vi "Interpolate 2D Scattered_Green Function.vi"(0 "X":dbl[](array[numeric]), 5 "Y":dbl[](array[numeric]), 7 "Z":dbl[](array[numeric]), 9 "Xi":dbl[](array[numeric]), 11 "Yi":dbl[](array[numeric])) -> (4 "Zi":dbl[](array[numeric]), 15 "error":i32)   [LabVIEW 2017, in "NI_AAL_Interpolation.lvlib"]
uses:
  <vilib>/gmath/NI_AAL_Interpolation.lvlib
  <vilib>/Analysis/7linalg.llb/Solve Linear Equations (single right hand).vi
  <vilib>/Analysis/baseanly.llb/Real Dot Product.vi
  <vilib>/Analysis/baseanly.llb/Solve Linear Equations By Cholesky.vi
  <vilib>/Analysis/baseanly.llb/Real Matrix to Compact Array.vi
  <vilib>/Analysis/baseanly.llb/Real Compact Tri-Matrix Linear Eqs.vi
  <vilib>/Analysis/7linalg.llb/Solve Linear Eqs (General).vi
  <vilib>/Analysis/7linalg.llb/Solve Linear Eqs (Gen, single right hand).vi
  <vilib>/Analysis/NI_AALPro.lvlib
  <vilib>/Analysis/NI_AALBase.lvlib
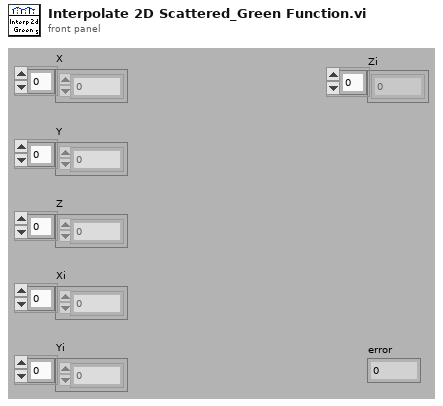
[diagram p1: front panel]
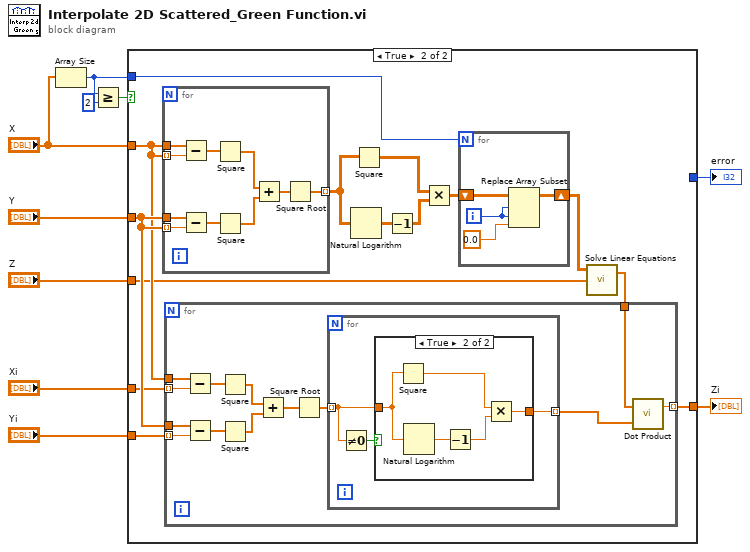
[diagram p0: block diagram]
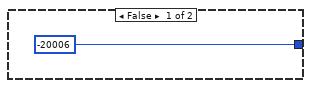
[diagram p2: hidden frame]
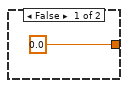
[diagram p3: hidden frame]
diagram:
  n1 = Array Size(array="X") -> (size(s)=w2:i32)
  n2 = Greater Or Equal?(x=w2, y=2) -> (x >= y?=w3:bool)
  n3 = case shown="True" w3 {
    tunnel: "Y" -> [_ w21]
    tunnel: "Xi" -> [_ w20]
    tunnel: "Yi" -> [_ w19]
    tunnel: "X" -> [_ w17]
    tunnel: "Z" -> [_ w16]
    tunnel: [_ w13] -> w6
    tunnel: w2 -> [_ w12]
    tunnel: [-20006 _] -> w1
    frame False {
    }
    frame True {
      n4 = for {
        tunnel: w17 -> [w61]
        tunnel: w21 -> [w60]
        tunnel: w17 -> [w59] mode=indexing
        tunnel: w21 -> [w58] mode=indexing
        tunnel: [w57] -> w25 mode=indexing
        n5 = Subtract(x=w61, y=w59) -> (x-y=w56:dbl[])
        n6 = Subtract(x=w60, y=w58) -> (x-y=w55:dbl[])
        n7 = Square(x=w56) -> (x^2=w53:dbl[])
        n8 = Square(x=w55) -> (x^2=w54:dbl[])
        n9 = Add(x=w53, y=w54) -> (x+y=w52:dbl[])
        n10 = Square Root(x=w52) -> (sqrt(x)=w57:dbl[])
      }
      n11 = Natural Logarithm(1:w25) -> (0:w24:dbl[][])
      n12 = Square(x=w25) -> (x^2=w22:dbl[][])
      n13 = Decrement(x=w24) -> (x-1=w23:dbl[][])
      n14 = Multiply(x=w22, y=w23) -> (x*y=w18:dbl[][])
      n15 = for {
        N: w12 -> [_]
        shift-right: [w28] -> w15
        shift-left: w18 -> [w29]
        i -> [w27]
        n16 = Replace Array Subset(array=w29, new element=0.0 ("new element/subarray"), index (row)=w27, index (col)=w27) -> (w28:dbl[][])
      }
      n17 = call-poly <vilib>:"Solve Linear Equations.vi"("Known Vector"=w16, "Input Matrix"=w15) -> ("Solution Vector"=w14:dbl[])  [unwired: 1 in, 1 out]
      n18 = for {
        tunnel: w17 -> [w42]
        tunnel: w21 -> [w40]
        tunnel: w20 -> [w41] mode=indexing
        tunnel: w19 -> [w39] mode=indexing
        tunnel: w14 -> [w31]
        tunnel: [w30] -> w13 mode=indexing
        n19 = Subtract(x=w42, y=w41) -> (x-y=w38:dbl[])
        n20 = Subtract(x=w40, y=w39) -> (x-y=w37:dbl[])
        n21 = Square(x=w38) -> (x^2=w36:dbl[])
        n22 = Square(x=w37) -> (x^2=w35:dbl[])
        n23 = Add(x=w36, y=w35) -> (x+y=w34:dbl[])
        n24 = Square Root(x=w34) -> (sqrt(x)=w33:dbl[])
        n25 = for {
          tunnel: w33 -> [w44] mode=indexing
          tunnel: [w43] -> w32 mode=indexing
          n26 = Not Equal To 0?(x=w44) -> (x != 0?=w45:bool)
          n27 = case shown="True" w45 {
            tunnel: w44 -> [_ w48]
            tunnel: [0.0 w47] -> w43
            frame False {
            }
            frame True {
              n28 = Square(x=w48) -> (x^2=w51:dbl)
              n29 = Natural Logarithm(1:w48) -> (0:w49:dbl)
              n30 = Decrement(x=w49) -> (x-1=w50:dbl)
              n31 = Multiply(x=w51, y=w50) -> (x*y=w47:dbl)
            }
          }
        }
        n32 = call-poly <vilib>:"Dot Product.vi"("Y Vector"=w32, "X Vector"=w31) -> ("X * Y"=w30:dbl)  [unwired: 1 out]
      }
    }
  }
  "Zi" <- w6
  "error" <- w1
